vi "Clear Interlock Alarm.vi"(8 "error in":errorcluster, 11 "6700 in":refnum<class "6700.lvclass">) -> (0 "error out":errorcluster, 3 "6700 out":refnum<class "6700.lvclass">)   [LabVIEW 2018, in "6700.lvlib" / "6700.lvclass"]
uses:
  6700.lvclass
  6700.lvclass/6700.ctl
  builds/Power_Supply.lvlibp/Power Supply.lvclass
  <instrlib>/Agilent N6700 Series/Agilent N6700 Series.lvlib
  C:/Users/Ron.Dexter.LUMINARTECH/Desktop/builds/Power_Supply.lvlibp/Power Supply.lvclass
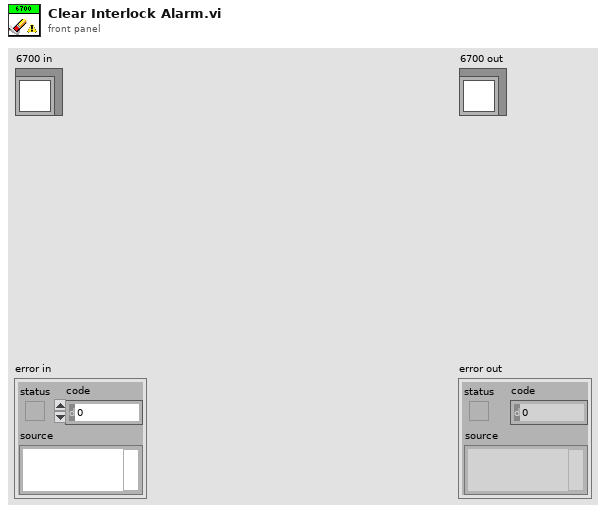
[diagram p1: front panel]
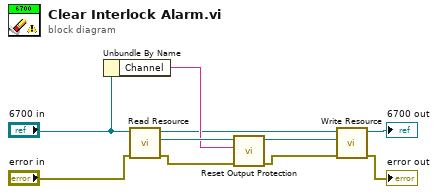
[diagram p0: block diagram]
diagram:
  n1 = Unbundle By Name("6700 in") -> ("Channel"=w2:string)
  n2 = call "Read Resource.vi"("error in"="error in", "Power Supply in"="6700 in") -> ("error out"=w3:errorcluster, "Resource"=w6:refnum<visa-resource-name>, "Power Supply out"=w1:refnum<class "6700.lvclass">)  [unwired: 7 in]
  n3 = call <instrlib>:"Reset Output Protection.vi"("error in (no error)"=w3, "Channel Name (1)"=w2, "VISA resource name"=w6) -> ("error out"=w4:errorcluster, "VISA resource name out"=w5:refnum<visa-resource-name>)  [unwired: 7 in]
  n4 = call "Write Resource.vi"("error in"=w4, "Resource"=w5, "Power Supply in"=w1) -> ("error out"=→"error out":errorcluster, "Power Supply out"=→"6700 out":refnum<class "6700.lvclass">)  [unwired: 7 in]
